vi "Disarm.vi"(8 "error in (no error)":errorcluster, 9 "Request type":T1, 10 "Requester":string, 11 "Pulse Recorder Actor in":refnum<class "Pulse Recorder Actor.lvclass">) -> (0 "error out":errorcluster, 3 "Pulse Recorder Actor out":refnum<class "Pulse Recorder Actor.lvclass">)   [LabVIEW 2021, in "Pulse Recorder Actor.lvclass"]
uses:
  Pulse Recorder Actor.lvclass
  Controllers/Process Controller/Request type.ctl
  Pulse Recorder Actor.lvclass/Pulse Recorder Actor.ctl
  Read Pulse driver.vi
  Write Pulse driver.vi
  NHMFL_Core/Libraries/Instruments/Pulse Driver/Pulse Driver.lvclass
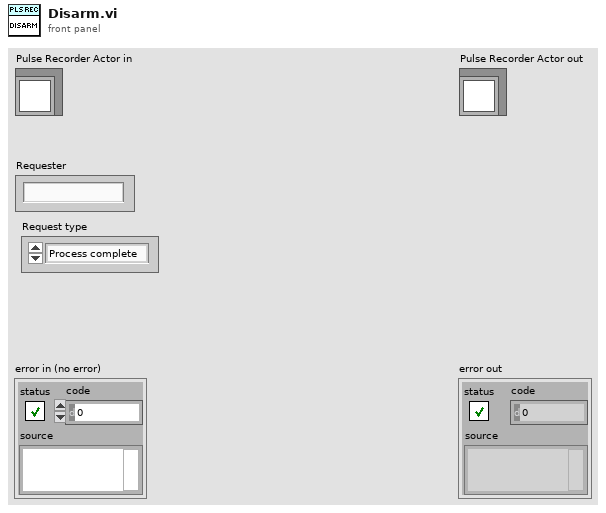
[diagram p1: front panel]
types:
  T1 = typedef "Request type.ctl" = enum16{"Process complete", "User command", "Auto-restart", "Error"}
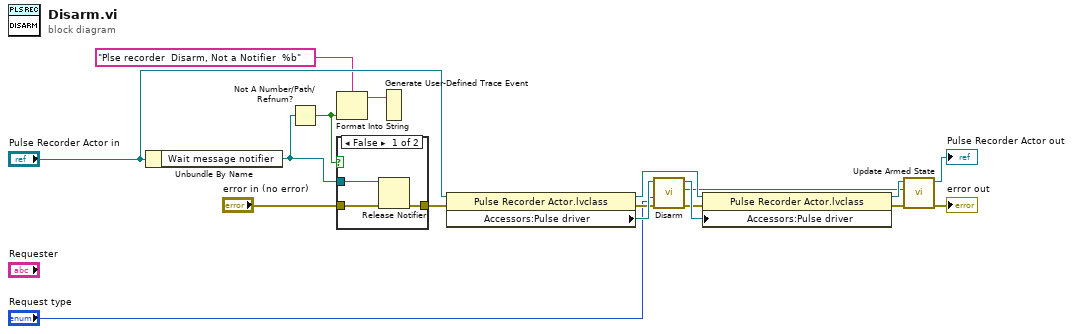
[diagram p0: block diagram]
diagram:
  n1 = Unbundle By Name("Pulse Recorder Actor in") -> ("Wait message notifier"=w10:refnum<notifier>)
  n2 = Not A Number/Path/Refnum?(number/path/refnum=w10) -> (NaN/Path/Refnum?=w2:bool)
  n3 = Format Into String(format string="Plse recorder  Disarm, Not a Notifier  %b" ("string"), w2) -> (resulting string=w4:string)  [unwired: 2 in, 1 out]
  n4 = case shown="False" w2 {
    tunnel: "error in (no error)" -> [w21 w22]
    tunnel: [w20 w22] -> w8
    tunnel: w10 -> [w19 _]
    frame False {
      n5 = Release Notifier(notifier=w19, error in (no error)=w21) -> (error out=w20:errorcluster)  [unwired: 1 in, 2 out]
    }
    frame True {
    }
  }
  n6 = Generate User-Defined Trace Event(2:w4) -> ()  [unwired: 1 in]
  n7 = property class="Pulse Recorder Actor.lvclass"(reference="Pulse Recorder Actor in", error in=w8) -> (reference out=w14:refnum<class "Pulse Recorder Actor.lvclass">, error out=w12:errorcluster, "Accessors:Pulse driver"=w16:refnum<class "Pulse Driver.lvclass">)
  n8 = call-dynamic "Disarm.vi"("error in (no error)"=w12, "Request type"="Request type", "Pulse Driver in"=w16) -> ("error out"=w11:errorcluster, "Armed"=w13:bool, "Pulse Driver out"=w15:refnum<class "Pulse Driver.lvclass">)  [unwired: 6 in]
  n9 = property class="Pulse Recorder Actor.lvclass"(reference=w14, error in=w11, "Accessors:Pulse driver"=w15) -> (reference out=w17:refnum<class "Pulse Recorder Actor.lvclass">, error out=w18:errorcluster)
  n10 = call-dynamic "Update Armed State.vi"("error in (no error)"=w18, "Armed"=w13, "Pulse Recorder in"=w17) -> ("error out"=→"error out":errorcluster, "Pulse Recorder out"=→"Pulse Recorder Actor out":refnum<class "Pulse Recorder Actor.lvclass">)  [unwired: 7 in]
